vi "Get Number of Points.vi"(8 "error in (no error)":errorcluster, 11 "Outline in":refnum<class "Outline.lvclass">) -> (0 "error out":errorcluster, 2 "Number of points":i32, 3 "Outline out":refnum<class "Outline.lvclass">)   [LabVIEW 2013, in "Outline.lvclass"]
uses:
  Outline.lvclass
  Outline.lvclass/Outline.ctl
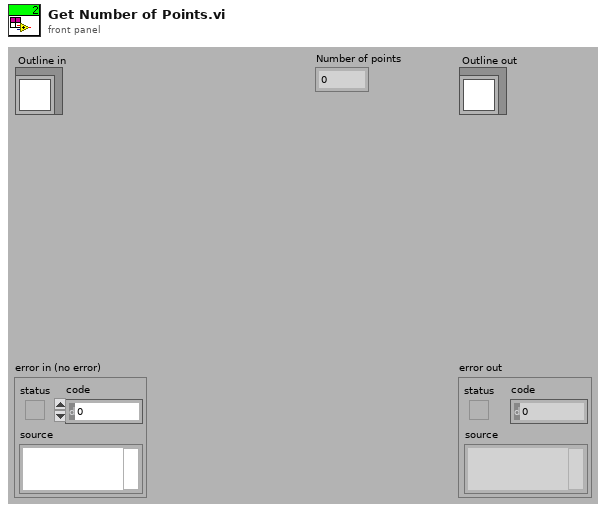
[diagram p1: front panel]
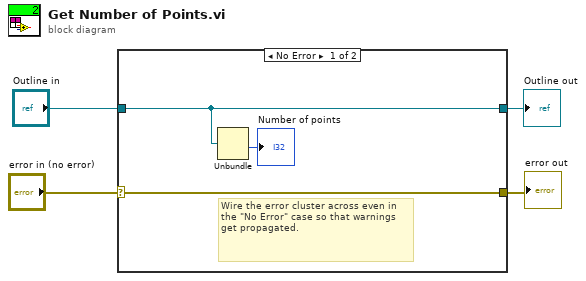
[diagram p0: block diagram]
diagram:
  n1 = case shown="No Error" "error in (no error)" {
    selector: "error in (no error)" -> [w7 w9]
    tunnel: [w7 w9] -> w3
    tunnel: [w6 w8] -> w1
    tunnel: "Outline in" -> [w6 w8]
    frame No Error {
      # "Wire the error cluster across even in the \"No Error\" case so that warnings get propagated."
      n2 = Unbundle(w6) -> (→"Number of points":i32)  [unwired: 3 out]
    }
    frame Error {
    }
  }
  "error out" <- w3
  "Outline out" <- w1
